vi "Offset_Gain_all_Ch.vi"() -> ()   [LabVIEW 2019]
uses:
  <userlib>/_TI-LA/Instr Drivers/Signal Generator/33XXX/Driver/EasyIO/Typedef/33XXX Standard Waveform Configuration.ctl
  <userlib>/_TI-LA/Instr Drivers/Signal Generator/33XXX/Driver/EasyIO/Typedef/33XXX Waveform Function.ctl
  <userlib>/_TI-LA/Instr Drivers/Signal Generator/33XXX/Driver/EasyIO/Typedef/33XXX Waveform Unit.ctl
  <userlib>/_TI-LA/Instr Drivers/Signal Generator/33XXX/Driver/EasyIO/Typedef/33XXX Output Load.ctl
  <userlib>/_TI-LA/Instr Drivers/Signal Generator/33XXX/Driver/EasyIO/Typedef/33XXX Output Load Termination.ctl
  <instrlib>/Agilent 34401/Public/Data/Read (Single Point).vi
  <vilib>/Analysis/NI_AALPro.lvlib
  <userlib>/_TI-LA/Instr Drivers/Signal Generator/33XXX/Driver/33XXX.lvlib
  <userlib>/_TI-LA/Instr Drivers/Signal Generator/33XXX/Modules/33XXX Modules.lvlib
  <instrlib>/Agilent 34401/Agilent 34401.lvlib
panel:
  out "Offset Error (mV)":dbl[](array[numeric])
  out "Gain Error (LSB)":dbl[](array[numeric])
  out "Measured Vref":dbl
  out "Mean[]":dbl[][](array[numeric])
  out "Intercept":dbl[](array[numeric])
  out "Slope":dbl[](array[numeric])
  in  "lv_scomp":u16=8
  in  "lv_ref_vol":u16
  in  "lv_ref_sel":u16
  in  "Standard Waveform Configuration":T1={"Frequency (Hz)"=1000.0, "Waveform Function"=1, "DC Offset (V)"=0.0, "Unit"=0, "Amplitude (V)"=1.0, "Duty cycle (%)"=50.0} {"Duty cycle (%)" min=0.002 max=99.999 step=0.001 format="%.3p"; "Amplitude (V)" min=0.001 max=20.0 format="%#_6p"; "Unit" items=["Vpp", "Vrms", "dB"]; "DC Offset (V)" min=-10.0 max=10.0 format="%#_6p"; "Waveform Function" items=["DC", "Sine", "Square", "Triangle", "Ramp", "Pulse", "Noise", "Sinc", "Negative Ramp", "Exponential Rise", "Exponential Fall", "Cardiac"]; "Frequency (Hz)" min=1e-06 max=80000000.0 format="%#_6p"}
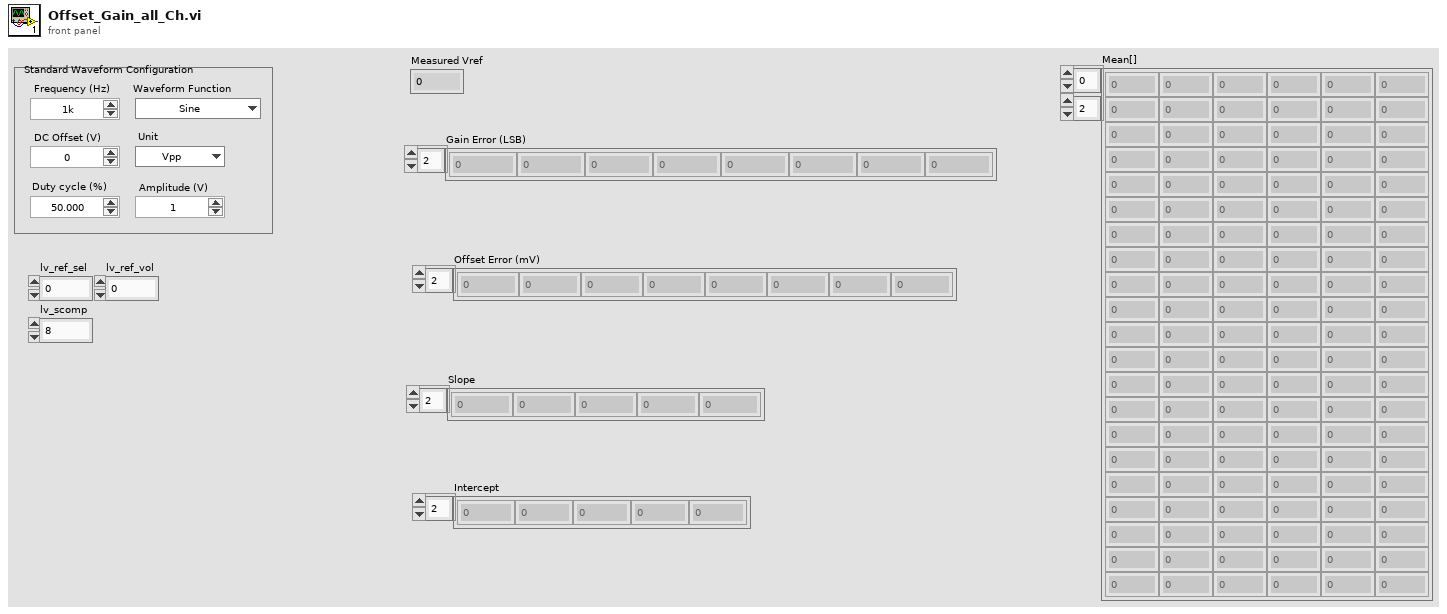
[diagram p1: front panel]
types:
  T1 = typedef "33XXX.lvlib/33XXX Standard Waveform Configuration.ctl" = cluster{"Frequency (Hz)":dbl, "Waveform Function":T2, "DC Offset (V)":dbl, "Unit":T3, "Amplitude (V)":dbl, "Duty cycle (%)":dbl}
  T2 = typedef "33XXX.lvlib/33XXX Waveform Function.ctl" = u16
  T3 = typedef "33XXX.lvlib/33XXX Waveform Unit.ctl" = u16
  T4 = typedef "33XXX.lvlib/33XXX Output Load.ctl" = cluster{"Output Load Impedence":T5, "Load value (ohms)":dbl}
  T5 = typedef "33XXX.lvlib/33XXX Output Load Termination.ctl" = enum16{"50 Ohms", "High Z", "User Defined"}
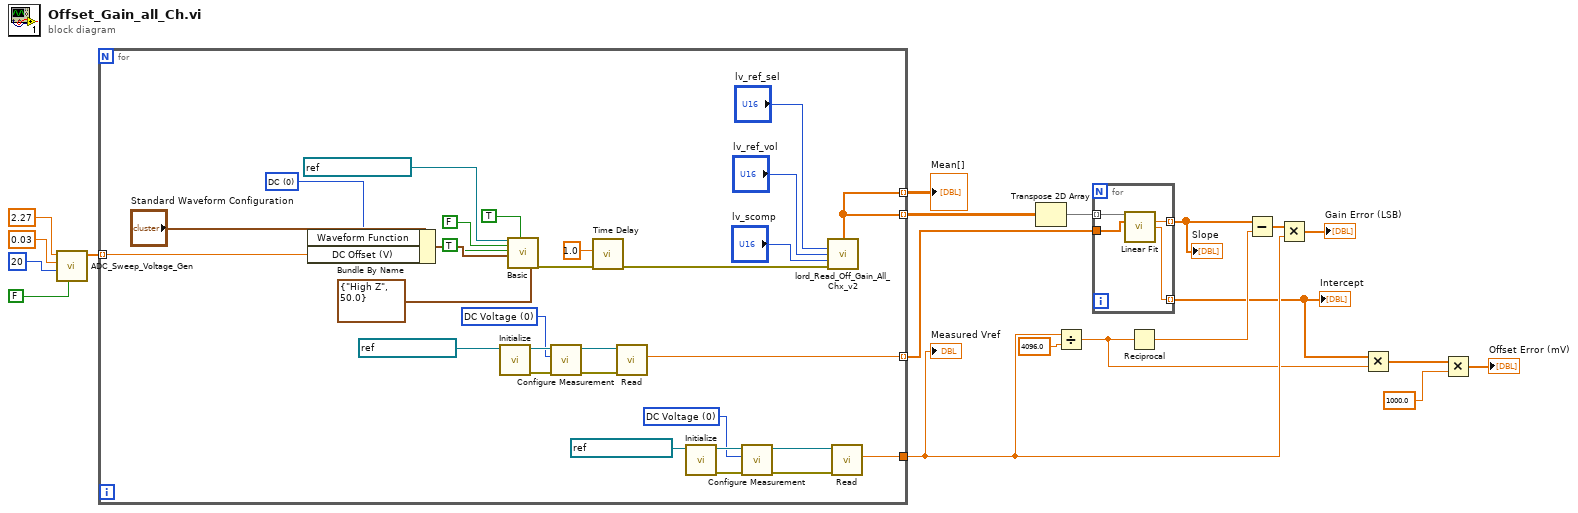
[diagram p0: block diagram]
diagram:
  n1 = call "ADC_Sweep_Voltage_Gen.vi"("Shuffle"=FALSE, "Count"=20, "Vn"=0.03, "Vp"=2.27) -> ("Vin_Array_Set"=w16:dbl[])  [unwired: 7 in]
  n2 = for {
    tunnel: w16 -> [w38] mode=indexing
    tunnel: [w22] -> w13 mode=indexing
    tunnel: [w36] -> w15 mode=indexing
    tunnel: [w36] -> w12 mode=indexing
    tunnel: [w23] -> w7
    w21 = T2 0 items=["DC", "Sine", "Square", "Triangle", "Ramp", "Pulse", "Noise", "Sinc", "Negative Ramp", "Exponential Rise", "Exponential Fall", "Cardiac"] ("Waveform Function")
    w24 = u16 0 items=["DC Voltage", "AC Voltage", "2 - Wire Resistance", "4 - Wire Resistance", "DC Current", "AC Current", "Frequency", "Period", "Continuity", "Diode Checking", "VDC:VDC Ratio", "Temperature", "Capacitance"] ("Function (0: DC Voltage)")
    w26 = u16 0 items=["DC Voltage", "AC Voltage", "2 - Wire Resistance", "4 - Wire Resistance", "DC Current", "AC Current", "Frequency", "Period", "Continuity", "Diode Checking", "VDC:VDC Ratio", "Temperature", "Capacitance"] ("Function (0: DC Voltage)")
    n3 = Bundle By Name(cluster="Standard Waveform Configuration", "Waveform Function"=w21, "DC Offset (V)"=w38) -> (w49:T1)
    n4 = call <instrlib>:"Initialize.vi"("VISA resource name"=refnum<visa-resource-name> "GPIB0::6::INSTR") -> ("error out"=w33:errorcluster, "VISA resource name out"=w32:refnum<visa-resource-name>)  [unwired: 9 in]
    n5 = call <userlib>:"Basic.vi"("Instrument Address"=refnum<visa-resource-name> "GPIB0::3::INSTR", "Reset?"=FALSE, "ID Query?"=TRUE, "Standard Waveform Configuration"=w49, "Enable Output?"=TRUE, "Output Load Configuration"=T4 {"Output Load Impedence"=enum."High Z", "Load value (ohms)"=50.0}) -> ("error out"=w40:errorcluster)  [unwired: 11 in, 2 out]
    n6 = call <instrlib>:"Configure Measurement.vi"("error in (no error)"=w33, "Function (0: DC Voltage)"=w24, "VISA resource name"=w32) -> ("error out"=w34:errorcluster, "VISA resource name out"=w35:refnum<visa-resource-name>)  [unwired: 7 in]
    n7 = call "Time Delay"("error in (no error)"=w40, "Delay Time (s)"=1.0) -> ("error out"=w44:errorcluster)  [unwired: 9 in]
    n8 = call-poly <instrlib>:"Read.vi"("error in (no error)"=w34, "VISA resource name"=w35) -> ("Measurement"=w22:dbl)  [unwired: 7 in, 2 out]
    n9 = call <instrlib>:"Initialize.vi"("VISA resource name"=refnum<visa-resource-name> "GPIB0::5::INSTR") -> ("error out"=w28:errorcluster, "VISA resource name out"=w30:refnum<visa-resource-name>)  [unwired: 9 in]
    n10 = call <instrlib>:"Configure Measurement.vi"("error in (no error)"=w28, "Function (0: DC Voltage)"=w26, "VISA resource name"=w30) -> ("error out"=w29:errorcluster, "VISA resource name out"=w31:refnum<visa-resource-name>)  [unwired: 7 in]
    n11 = call "lord_Read_Off_Gain_All_Chx_v2.vi"("lv_ref_sel"="lv_ref_sel", "lv_ref_vol"="lv_ref_vol", "lv_scomp"="lv_scomp", "error in"=w44) -> ("Mean[]"=w36:dbl[])  [unwired: 3 in, 8 out]
    n12 = call-poly <instrlib>:"Read.vi"("error in (no error)"=w29, "VISA resource name"=w31) -> ("Measurement"=w23:dbl)  [unwired: 7 in, 2 out]
  }
  "Mean[]" <- w12
  "Measured Vref" <- w7
  n13 = Transpose 2D Array(2D array=w15) -> (transposed array=w14:dbl[][])
  n14 = Divide(x=w7, y=4096.0) -> (x/y=w4:dbl)
  n15 = for {
    tunnel: w14 -> [w54] mode=indexing
    tunnel: w13 -> [w53]
    tunnel: [w52] -> w10 mode=indexing
    tunnel: [w51] -> w5 mode=indexing
    n16 = call <vilib>:"Linear Fit.vi"("Y"=w54, "X"=w53) -> ("slope"=w52:dbl, "intercept"=w51:dbl)  [unwired: 9 in, 3 out]
  }
  "Slope" <- w10
  "Intercept" <- w5
  n17 = Reciprocal(x=w4) -> (1/x=w9:dbl)
  n18 = Subtract(x=w10, y=w9) -> (x-y=w8:dbl[])
  n19 = Multiply(x=w8, y=w7) -> (x*y=→"Gain Error (LSB)":dbl[])
  n20 = Multiply(x=w5, y=w4) -> (x*y=w3:dbl[])
  n21 = Multiply(x=w3, y=1000.0) -> (x*y=→"Offset Error (mV)":dbl[])
